vi "Generate BER Curve.vi"(4 "M-PSK":i32=16, 5 "Samples":i32=30, 6 "Sample Step":dbl=1.0, 7 "Averaging Number":i32=100, 8 "Initial Value":i32, 9 "Message Bits":i32=500, 10 "Synchronization Sequence":i32=40, 11 "Zero Pad":i32=40) -> (0 "error out":errorcluster, 1 "Current Value":dbl, 2 "BER Curve":dbl[](array[numeric]), 3 "Waveform Graph":dbl[](graph))   [LabVIEW 2013]
uses:
  <vilib>/addons/Modulation/Digital/General/MT Generate PSK System Parameters(M).vi
  <vilib>/addons/Modulation/Digital/General/MT Generate Bits (Galois, PN Order).vi
  <vilib>/addons/Modulation/Digital/General/MT Generate PSK Synchronization Parameters (bit array).vi
  <vilib>/addons/Modulation/niDMT.lvlib
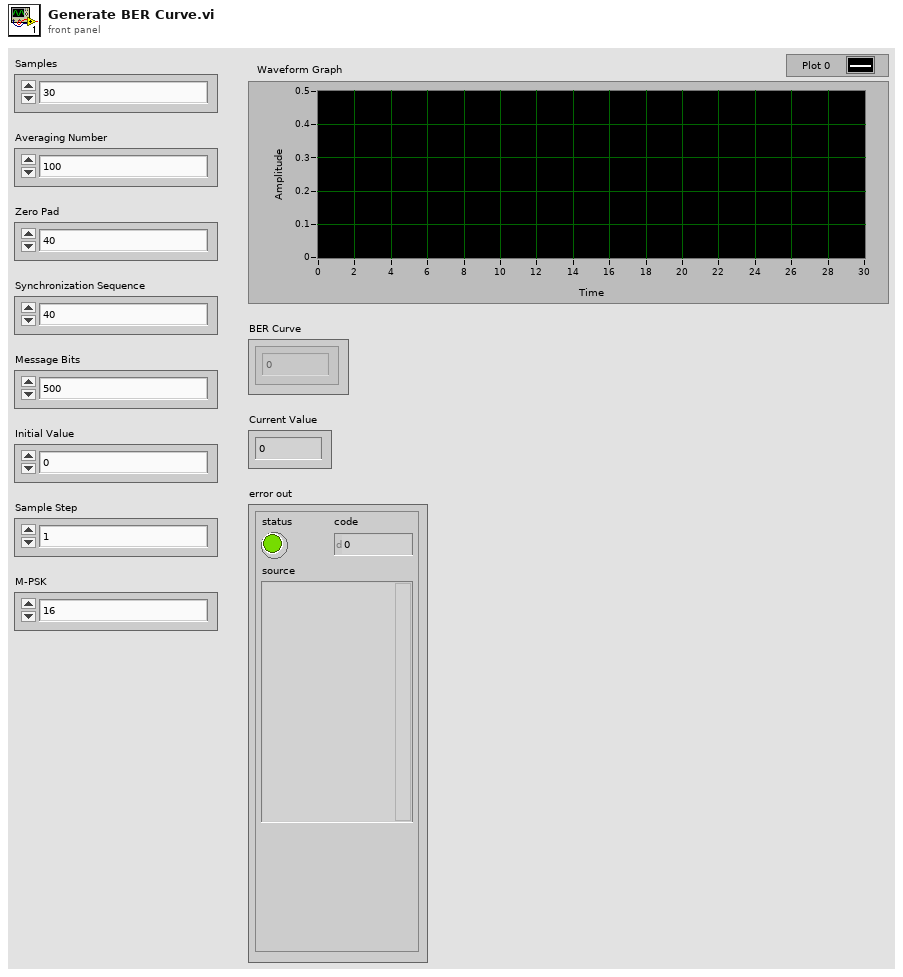
[diagram p1: front panel]
types:
  T1 = enum16{"FSK", "PSK", "QAM", "MSK", "PAM", "ASK", "CPM"}
  T2 = enum16{"none", "Raised Cosine", "Root Raised Cos", "Gaussian"}
  T3 = cluster{"samples per symbol (16)":i32, "symbol map":cdb[], "differential PSK":enum16{"disable", "enable"}, "PSK type":u16}
  T4 = typedef "niAMT.lvlib/Complex Data Waveform.ctl" = cluster{"t0":dbl, "dt":dbl, "Y":cdb[]}
  T5 = cluster{"expected sync location (symbols)":i32, "sync sequence":cdb[], "sync location uncertainty (symbols)":i32, "sync indent (symbols)":i32}
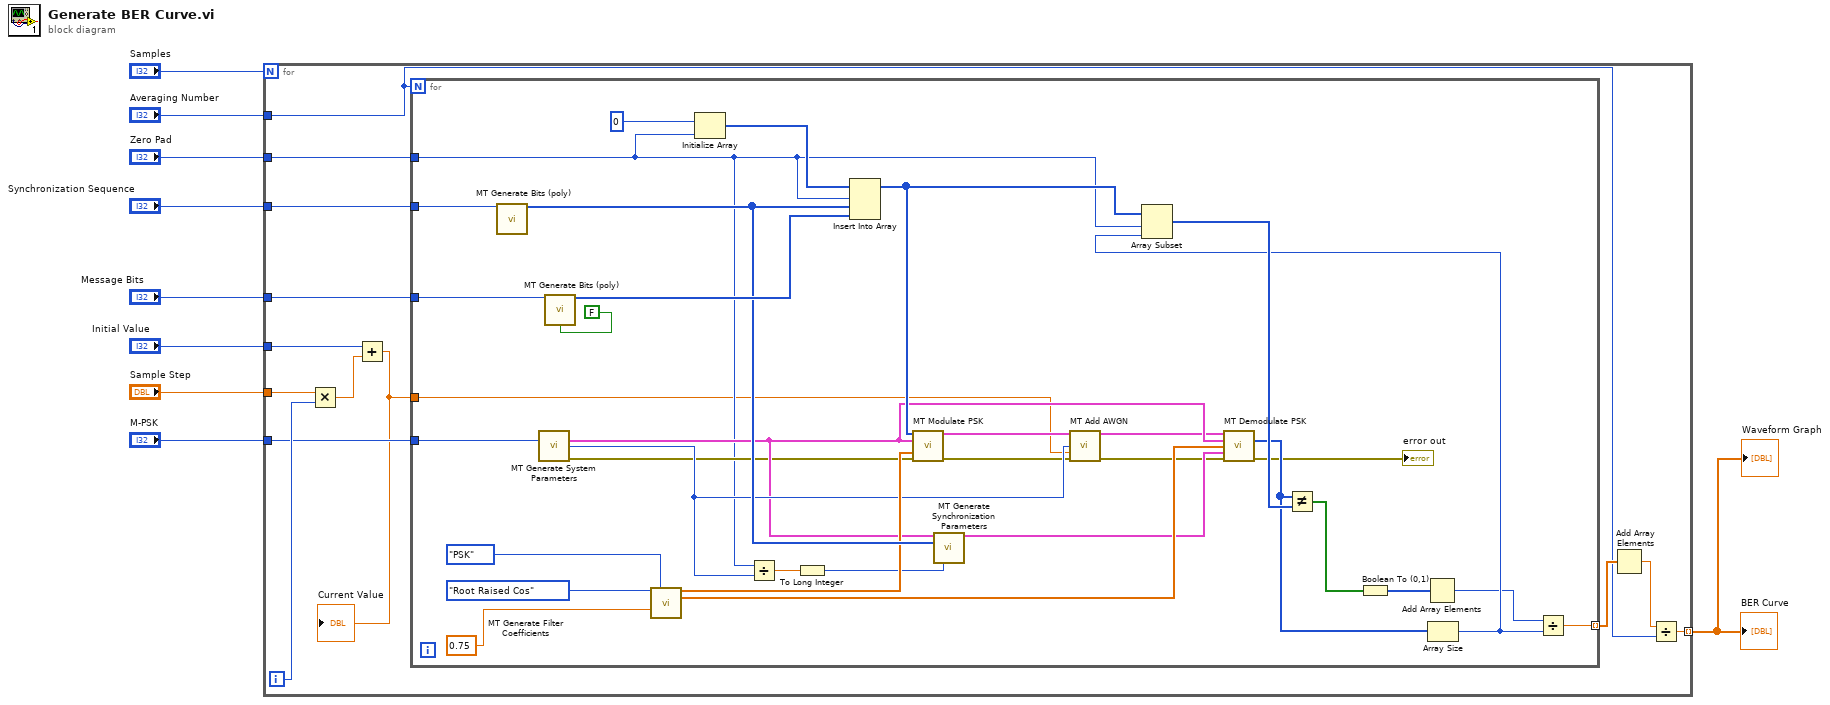
[diagram p0: block diagram]
diagram:
  n1 = for {
    N: "Samples" -> [_]
    tunnel: "Sample Step" -> [w21]
    tunnel: "Zero Pad" -> [w18]
    tunnel: "M-PSK" -> [w15]
    tunnel: [w13] -> w6 mode=indexing
    tunnel: "Initial Value" -> [w20]
    tunnel: "Message Bits" -> [w16]
    tunnel: "Synchronization Sequence" -> [w17]
    tunnel: "Averaging Number" -> [w11]
    i -> [w22]
    n2 = Multiply(x=w21, y=w22) -> (x*y=w19:dbl)
    n3 = Add(x=w20, y=w19) -> (x+y=w10:dbl)
    "Current Value" <- w10
    n4 = for {
      N: w11 -> [_]
      tunnel: w18 -> [w28]
      tunnel: w17 -> [w27]
      tunnel: w16 -> [w26]
      tunnel: w10 -> [w25]
      tunnel: [w24] -> w14 mode=indexing
      tunnel: w15 -> [w23]
      n5 = call-poly <vilib>:"MT Generate Bits (poly).vi"("total bits (128)"=w27) -> ("output bit stream"=w54:i8[])  [unwired: 12 in, 2 out]
      n6 = call-poly <vilib>:"MT Generate System Parameters.vi"("M-PSK (4)"=w23) -> ("PSK system parameters"=w37:T3, "bits per symbol"=w41:i32, "error out"=w32:errorcluster)  [unwired: 12 in]
      n7 = call-poly <vilib>:"MT Generate Bits (poly).vi"("total bits (128)"=w26, "reset? (T)"=FALSE) -> ("output bit stream"=w56:i8[])  [unwired: 11 in, 2 out]
      n8 = call <vilib>:"MT Generate Filter Coefficients.vi"("pulse shaping filter (none)"=T2."Root Raised Cos", "modulation type"=T1."PSK", "filter parameter"=0.75) -> ("pulse shaping filter coefficients"=w42:dbl[], "matched filter coefficients"=w43:dbl[])  [unwired: 10 in, 1 out]
      n9 = Initialize Array "Initialize Array"(0, w28) -> (w30:i32[])
      n10 = Divide(x=w28, y=w41) -> (x/y=w39:dbl)
      n11 = To Long Integer(number=w39) -> (32bit integer=w40:i32)
      n12 = Insert Into Array "Insert Into Array"(array=w30, index=w28, new element #1=w54, new element #2=w56) -> (w51:i32[])
      n13 = call <vilib>:"MT Modulate PSK.vi"("input bit stream"=w51, "PSK system parameters"=w37, "pulse shaping filter coefficients"=w42, "error in (no error)"=w32) -> ("output complex waveform"=w33:T4, "error out"=w34:errorcluster)  [unwired: 9 in, 1 out]
      n14 = call-poly <vilib>:"MT Generate Synchronization Parameters.vi"("PSK system parameters"=w37, "sync bits"=w54, "expected sync location (symbols)"=w40) -> ("PSK synchronization parameters"=w38:T5)  [unwired: 11 in, 1 out]
      n15 = call <vilib>:"MT Add AWGN.vi"("input complex waveform"=w33, "bits per symbol (1)"=w41, "Eb/N0 (10 dB)"=w25, "error in (no error)"=w34) -> ("output complex waveform"=w36:T4, "error out"=w35:errorcluster)  [unwired: 9 in, 1 out]
      n16 = call <vilib>:"MT Demodulate PSK.vi"("input complex waveform"=w36, "PSK system parameters"=w37, "matched filter coefficients"=w43, "synchronization parameters"=w38, "error in (no error)"=w35) -> ("output bit stream"=w50:i8[], "error out"=→"error out":errorcluster)  [unwired: 6 in, 3 out]
      n17 = Array Size(array=w50) -> (size(s)=w52:i32)
      n18 = Array Subset "Array Subset"(array=w51, index=w28, length=w52) -> (w53:i32[])
      n19 = Not Equal?(x=w50, y=w53) -> (x != y?=w47:bool[])
      n20 = Boolean To (0,1)(Boolean=w47) -> (0, 1=w48:i16[])
      n21 = Add Array Elements(numeric array=w48) -> (sum=w46:i16)
      n22 = Divide(x=w46, y=w52) -> (x/y=w24:dbl)
    }
    n23 = Add Array Elements(numeric array=w14) -> (sum=w12:dbl)
    n24 = Divide(x=w12, y=w11) -> (x/y=w13:dbl)
  }
  "BER Curve" <- w6
  "Waveform Graph" <- w6
